vi "FadeColor.vi"(6 "Reset":bool, 9 "FadeRate":u32, 10 "FadeColor in":fxp<+,3,3>, 11 "Color in":fxp<+,3,3>) -> (3 "FadeColor out":fxp<+,3,3>)   [LabVIEW 2019, in "GameEngine.lvlib"]
uses:
  GameEngine.lvlib
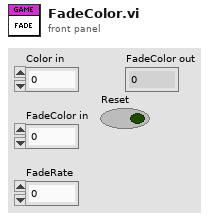
[diagram p1: front panel]
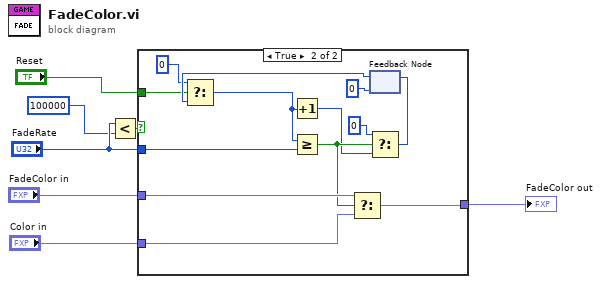
[diagram p0: block diagram]
diagram:
  n1 = Less?(x="FadeRate", y=u32 100000) -> (x < y?=w4:bool)
  n2 = case shown="True" w4 {
    tunnel: "FadeColor in" -> [_ w21]
    tunnel: [w8 w19] -> w6
    tunnel: "FadeRate" -> [_ w18]
    tunnel: "Color in" -> [w8 w12]
    tunnel: "Reset" -> [_ w9]
    frame False {
    }
    frame True {
      n3 = feedback #1(u32 0 ("x")) -> (w17:u32)
      n4 = Select(t=u32 0 ("f"), s=w9, f=w17) -> (s? t:f=w11:u32)
      n5 = Increment(x=w11) -> (x+1=w14:u32)
      n6 = Greater Or Equal?(x=w11, y=w18) -> (x >= y?=w20:bool)
      n7 = Select(t=w21, s=w20, f=w12) -> (s? t:f=w19:fxp<+,3,3>)
      n8 = Select(t=u32 0, s=w20, f=w14) -> (s? t:f=w15:u32)
      n9 = feedback-in #1(w15) -> ()
    }
  }
  "FadeColor out" <- w6
